vi "getPhaseMeasurement.vi"(8 "error in (no error)":errorcluster, 9 "Source 2":string, 10 "Source 1":string, 11 "Scope in":refnum<class "Scope.lvclass">) -> (0 "error out":errorcluster, 2 "Numeric":dbl, 3 "Scope out":refnum<class "Scope.lvclass">)   [LabVIEW 2023, in "sweScope.lvlib" / "Scope.lvclass"]
doc: "<b>Author:</b> Wolfgang\n<b>Descritpion:</b> Measure the phase shift between two sources."
uses:
  Scope.lvclass
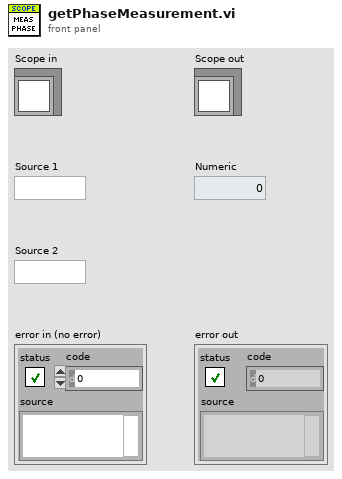
[diagram p1: front panel]
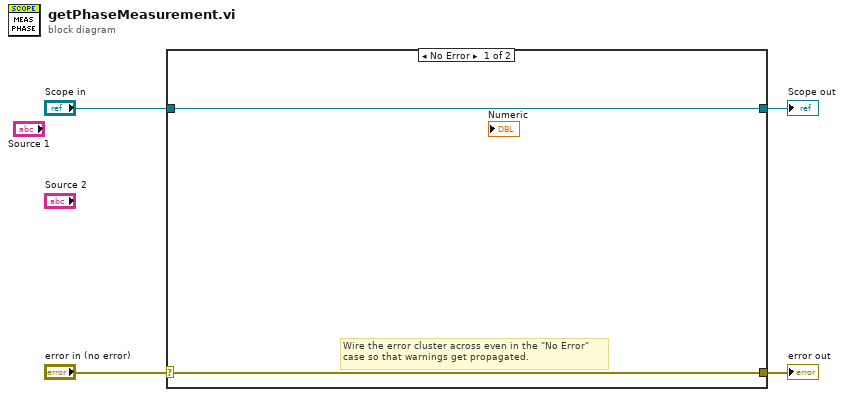
[diagram p0: block diagram]
diagram:
  n1 = case shown="No Error" "error in (no error)" {
    selector: "error in (no error)" -> [w5 w8]
    tunnel: [w5 w8] -> w3
    tunnel: [w6 w7] -> w1
    tunnel: "Scope in" -> [w6 w7]
    frame No Error {
      # "Wire the error cluster across even in the \"No Error\"\ncase so that warnings get propagated."
    }
    frame Error {
    }
  }
  "error out" <- w3
  "Scope out" <- w1
